vi "Oxford-VRM-Main-Launcher.vi"() -> ()   [LabVIEW 2016]
doc: "This VI will launch the PPMS 2 Instrument backend that will contunously monitor the state of the instrument and log to the DSC. The user has the option of launching a user interface (default) or allowing the backend to run headless. Run \"Launch PPMS2 UI.vi\" here or on a different computer to have a remote user interface. You can also use the APIs like \"Get Temperturature\" interact programmatically with the PPMS 2 Instrument backend."
uses:
  <vilib>/JKI/JKI SMO/SMO/SMO.lvclass
  <vilib>/JKI/JKI SMO/SMO/Typedefs/SMOState --Enum.ctl
  <vilib>/JKI/JKI SMO/SMO.UI/SMO.UI.lvclass
  <userlib>/LevyLab/Levylab Instruments/SMOs/Instrument UI/Instrument UI.lvclass
  SMOs/Instrument.OxfordVRM UI/Instrument.OxfordVRM UI.lvclass
  SMOs/Instrument.OxfordVRM/Instrument.OxfordVRM.lvclass
  C:/Program Files (x86)/National Instruments/LabVIEW 2016/vi.lib/JKI/JKI SMO/SMO/SMO.lvclass
  C:/Program Files (x86)/National Instruments/LabVIEW 2016/user.lib/LevyLab/Levylab Instruments/SMOs/Instrument/Instrument.lvclass
  C:/Program Files (x86)/National Instruments/LabVIEW 2016/vi.lib/JKI/JKI SMO/SMO.UI/SMO.UI.lvclass
  C:/Program Files (x86)/National Instruments/LabVIEW 2016/user.lib/LevyLab/Levylab Instruments/SMOs/Instrument UI/Instrument UI.lvclass
panel:
  in  "Debug Mode?":bool
  in  "Stop":bool=TRUE
  in  "Start":bool=TRUE
  in  "Splash Status":string="Push Start to Start..." caption="String"
  out "UI SMO State":T1=enum."Stopped"
  out "SMO State":T1
  out "error out":errorcluster
  # "OI 1820"
  # "v"
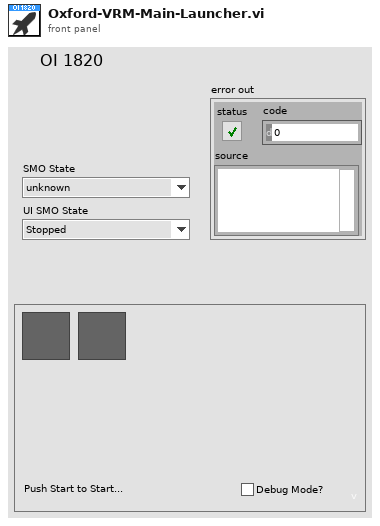
[diagram p1: front panel]
types:
  T1 = typedef "SMO.lvclass/SMOState --Enum.ctl" = enum16{"unknown", "Created", "Started", "Stopped"}
  T2 = enum32{"Invalid", "Standard", "Closed", "Hidden", "Minimized", "Maximized"}
  T3 = enum32{"invalid app kind", "Development System", "Run Time System", "Student Edition", "Embedded LabVIEW", "Evaluation", "Custom"}
  T4 = cluster{"Core":cluster{"Current VI Reference":refnum<vi>, "Close Panel on Exit?":bool}, "Instrument.OxfordVRM":refnum<class "Instrument.OxfordVRM.lvclass">, "Instrument.OxfordVRM UI":refnum<class "Instrument.OxfordVRM UI.lvclass">}
  T5 = cluster{"Current VI Reference":refnum<vi>, "Close Panel on Exit?":bool}
  T6 = typedef "SMO.lvclass/Public Events.ctl" = cluster{"Error":refnum<user-event>, "State":refnum<user-event>, "Reserve State":refnum<user-event>}
  T7 = typedef "SMO.UI.lvclass/PublicEvents--Cluster.ctl" = cluster{"UI Hidden":refnum<user-event>, "UI State":refnum<user-event>}
  T8 = cluster{"Event Registration Refnum":refnum<event-registration>, "Event Registration Refnum":refnum<event-registration>}
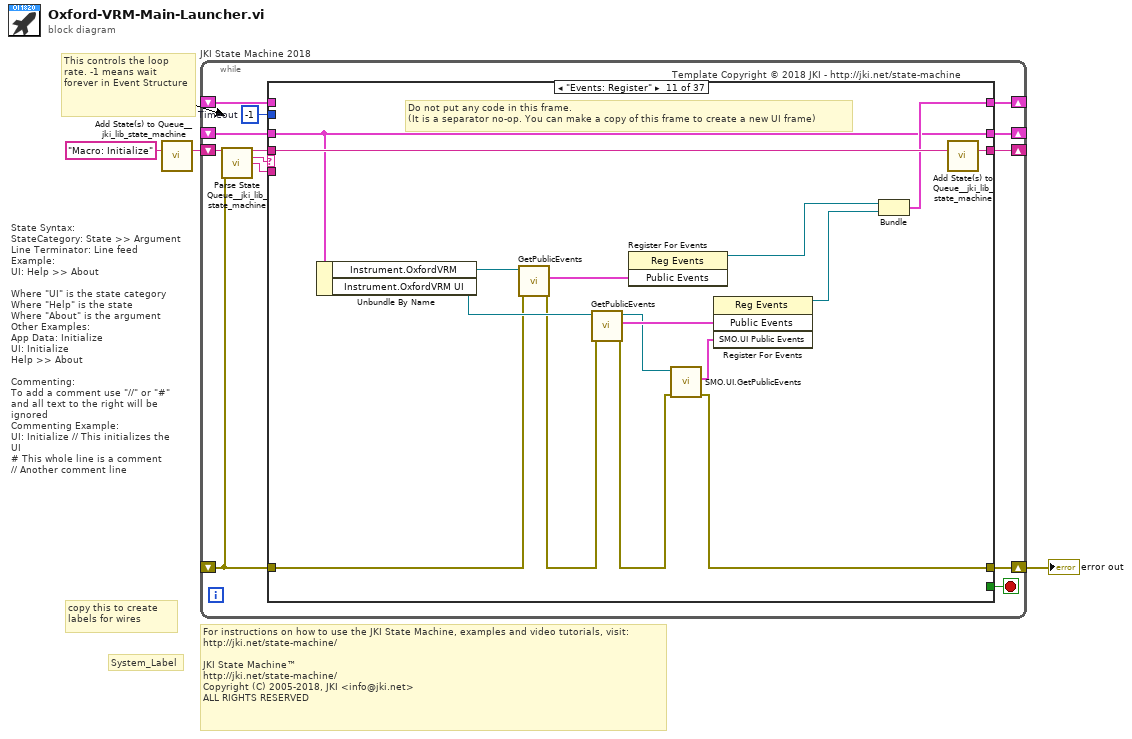
[diagram p0: block diagram]
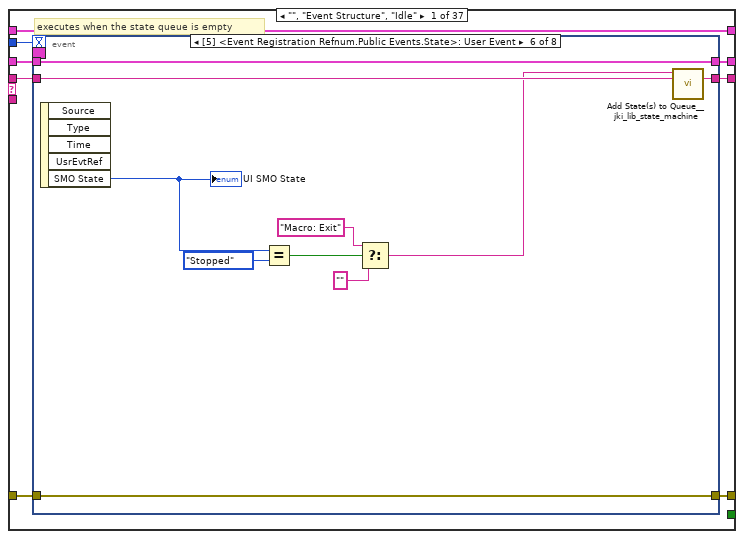
[diagram p2: hidden frame]
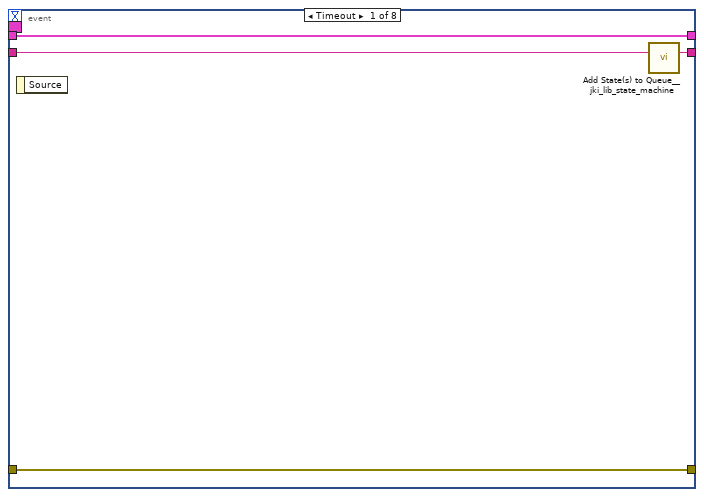
[diagram p3: hidden frame]
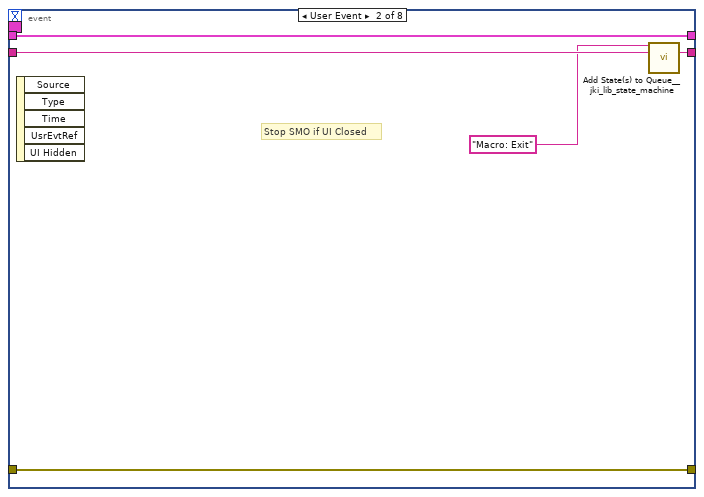
[diagram p4: hidden frame]
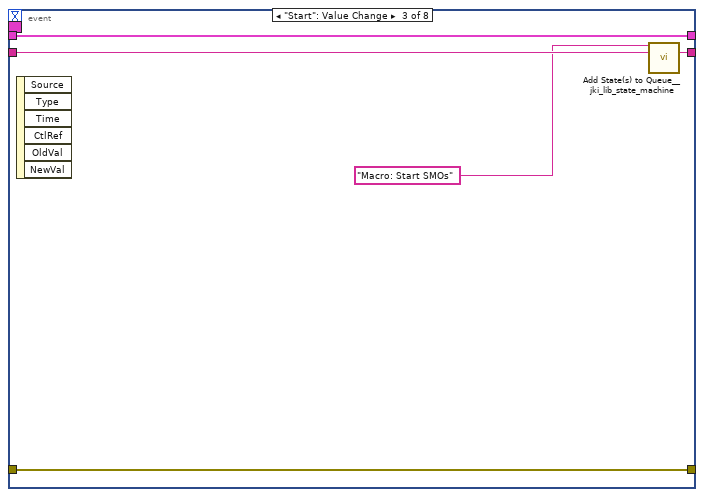
[diagram p5: hidden frame]
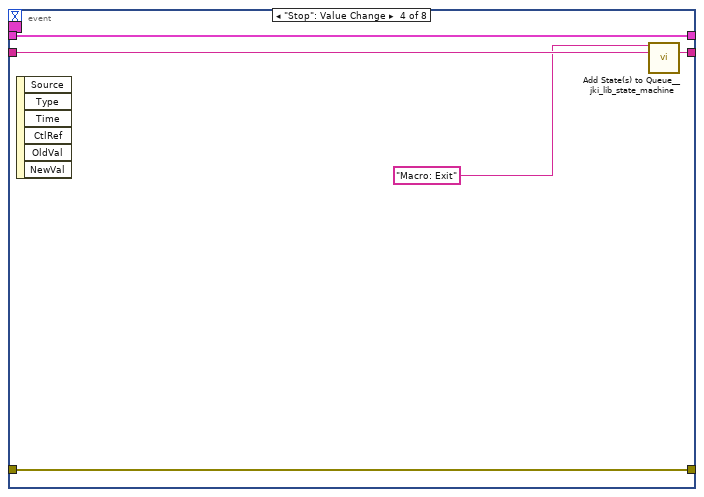
[diagram p6: hidden frame]
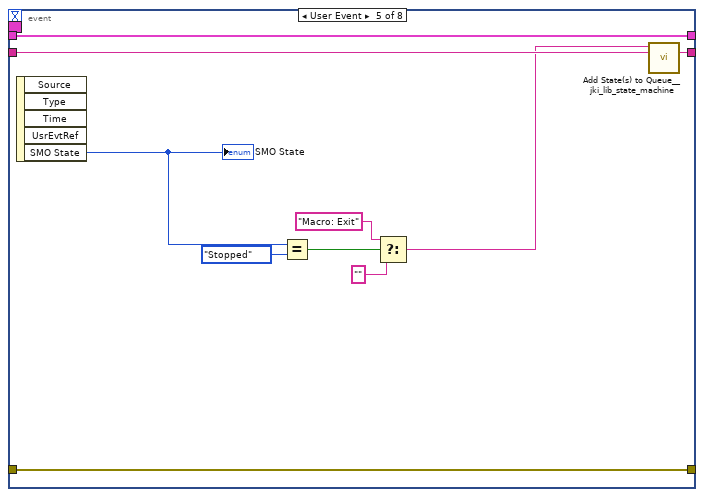
[diagram p7: hidden frame]
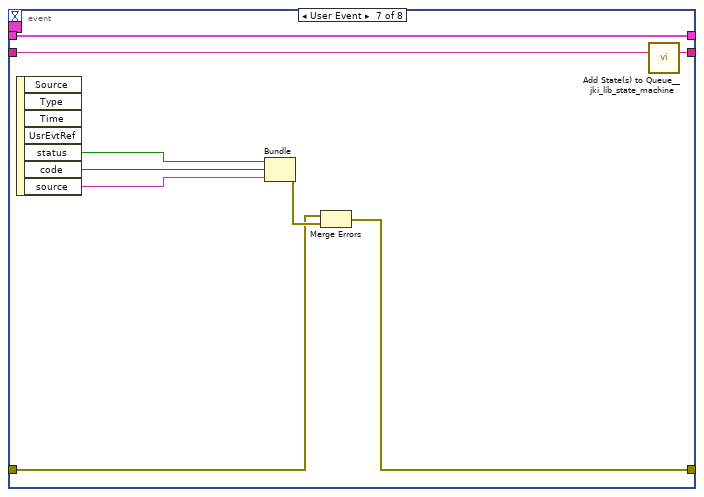
[diagram p8: hidden frame]
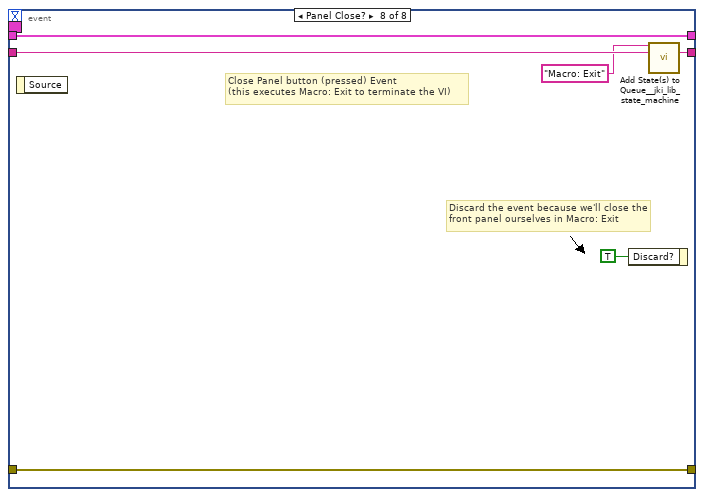
[diagram p9: hidden frame]
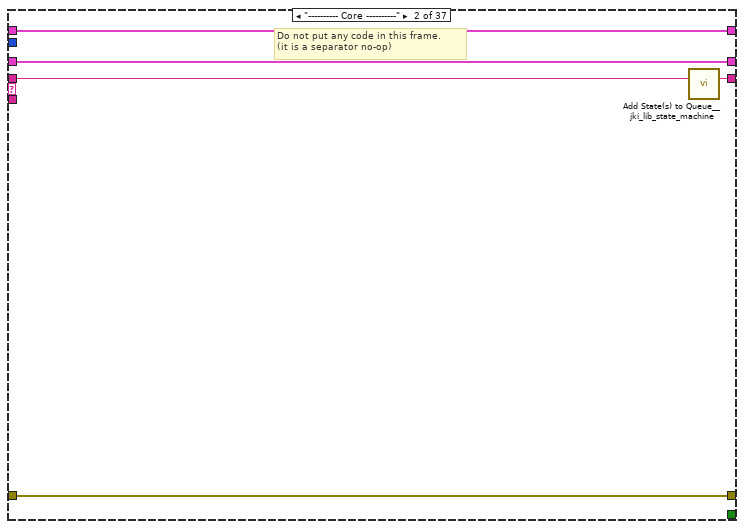
[diagram p10: hidden frame]
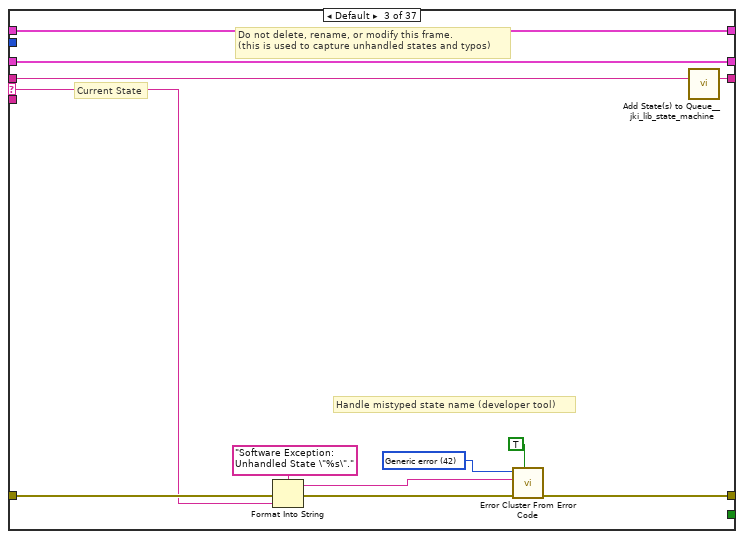
[diagram p11: hidden frame]
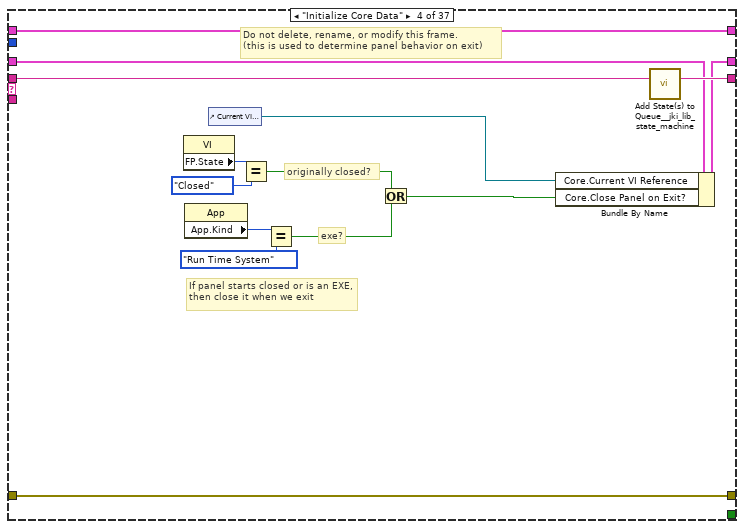
[diagram p12: hidden frame]
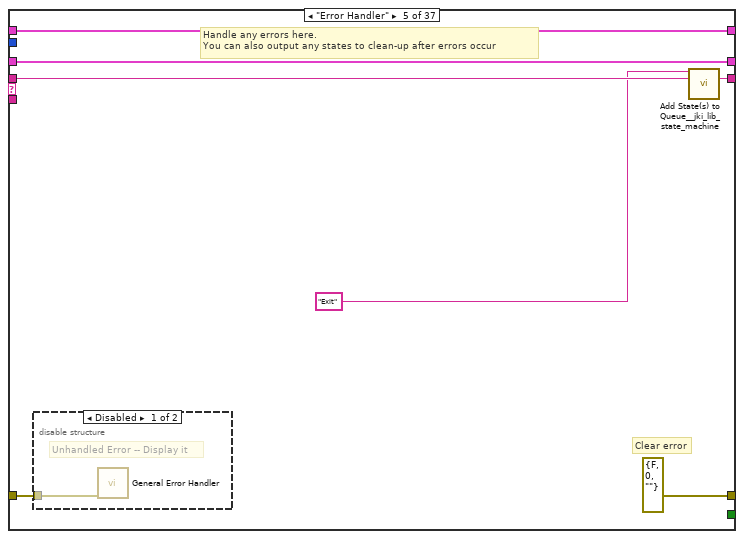
[diagram p13: hidden frame]
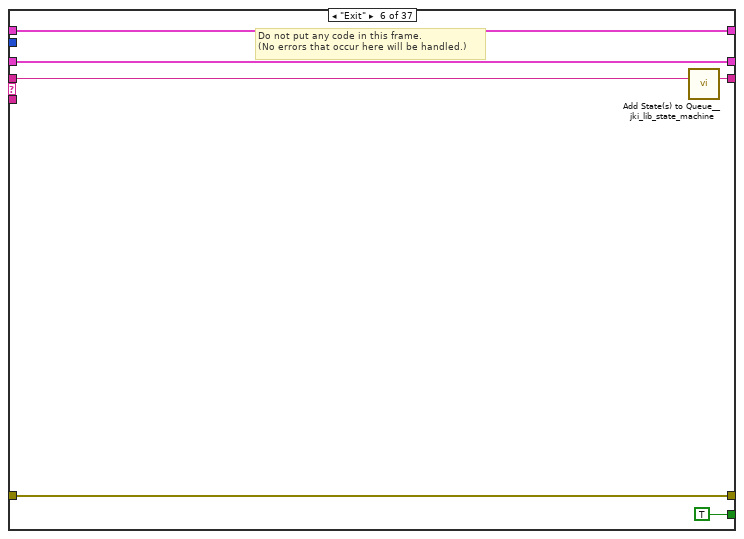
[diagram p15: hidden frame]
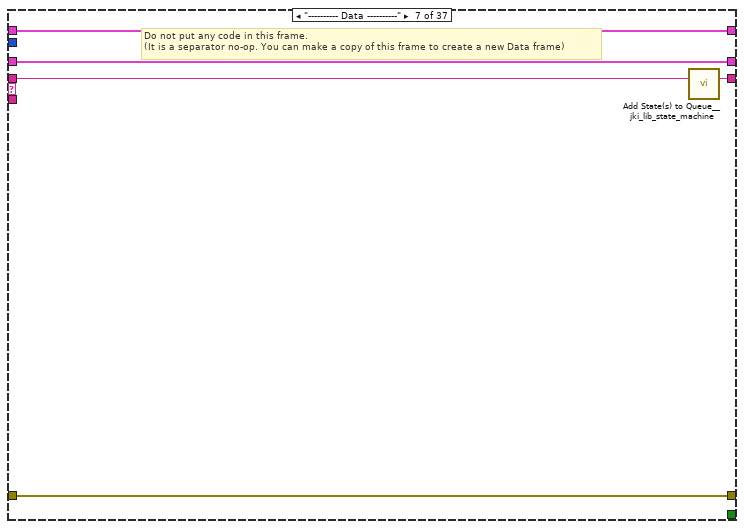
[diagram p16: hidden frame]
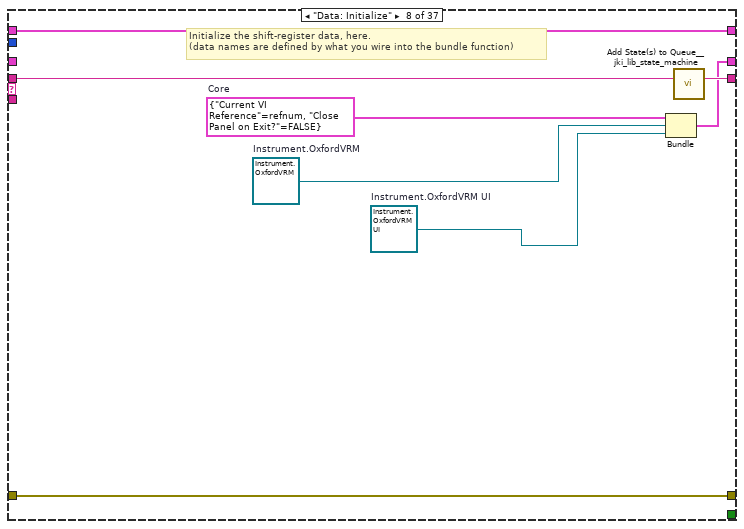
[diagram p17: hidden frame]
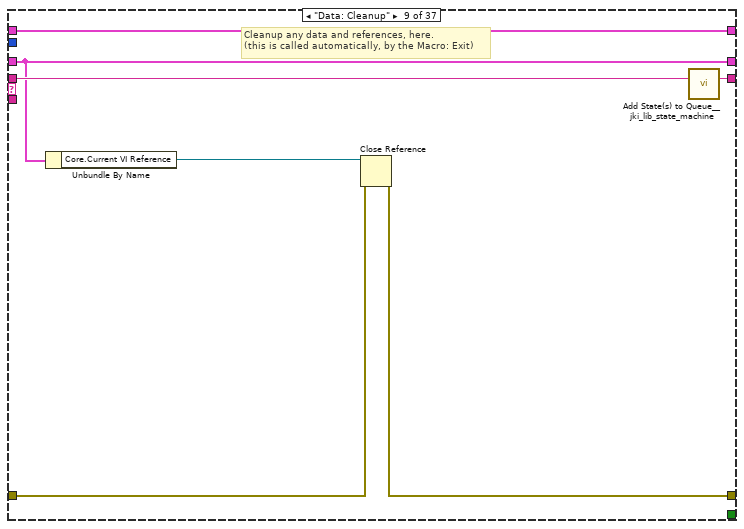
[diagram p18: hidden frame]
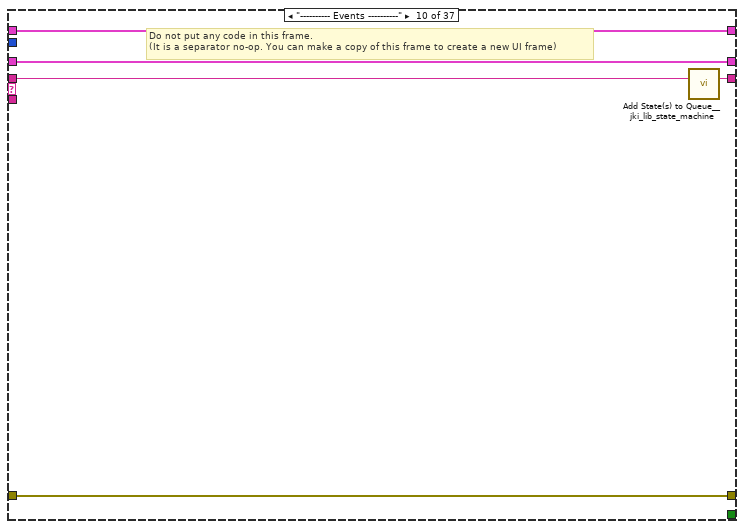
[diagram p19: hidden frame]
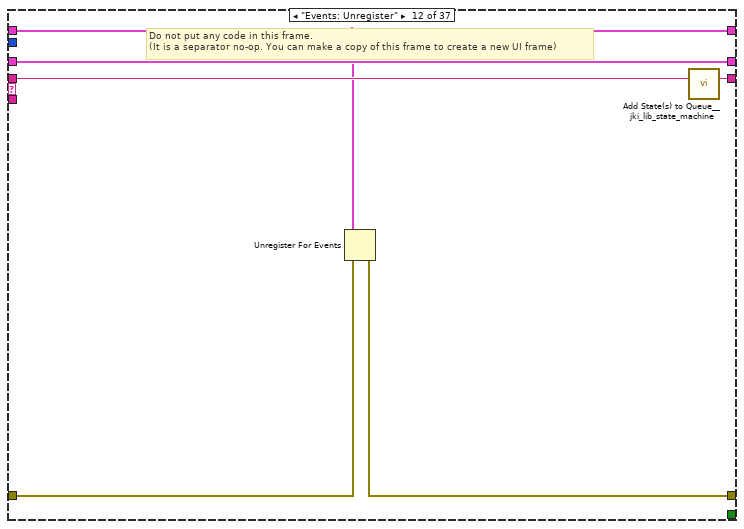
[diagram p20: hidden frame]
diagram:
  # "For instructions on how to use the JKI State Machine, examples and video tutorials, visit:\nhttp://jki.net/state-machine/\n\nJKI State Machine™\nhttp://jki.net/state-machine/\nCopyright (C) 2005-2018, JKI <info@jki.net>\nALL RIGHTS RESERVED"
  # "State Syntax:\nStateCategory: State >> Argument\nLine Terminator: Line feed\nExample:\nUI: Help >> About\n\nWhere \"UI\" is the state category\nWhere \"Help\" is the state\nWhere \"About\" is the argument\nOther Examples:\nApp Data: Initialize\nUI: Initialize\nHelp >> About\n\nCommenting:\nTo add a comment use \"//\" or \"#\" and all text to the right will be ignored\nCommenting Example:\nUI: Initialize // This initializes the UI\n# This whole line is a comment\n// Another comment line"
  # "copy this to create labels for wires"
  # "This controls the loop rate. -1 means wait forever in Event Structure"
  # "System_Label"
  n1 = call <vilib>:"Add State(s) to Queue__jki_lib_state_machine.vi"("State(s) in (\"\")"="Macro: Initialize") -> ("States Out"=w3:string)  [unwired: 14 in]
  n2 = while "JKI State Machine 2018" {
    shift-right: [w9] -> _
    shift-left: _ -> [w4]
    shift-right: [w12] -> w1
    shift-left: _ -> [w7]
    shift-right: [w11] -> _
    shift-left: w3 -> [w13]
    shift-right: [w6] -> _
    shift-left: _ -> [w5]
    stop <- w10 stop-if-true
    w8 = -1  # Timeout
    # "Template Copyright © 2018 JKI - http://jki.net/state-machine"
    n3 = call <vilib>:"Parse State Queue__jki_lib_state_machine.vi"("State Queue"=w13, "Error In (no error)"=w7) -> ("Remaining States"=w15:string, "Current State"=w16:string, "Arguments"=w14:string)  [unwired: 11 in]
    n4 = case shown="\"Events: Register\"" w16 {
      selector: w16 -> [_ _ w85 _ _ _ _ _ _ _ _ _ _ _ _ _ _ _ _ _ _ _ _ _ _ _ _ _ _ _ _ _ _ _ _ _ _]
      tunnel: w15 -> [w24 w83 w89 w109 w116 w123 w128 w136 w143 w148 w164 w170 w175 w181 w188 w200 w278 w283 w288 w294 w300 w306 w318 w323 w337 w346 w357 w372 w386 w393 w404 w419 w434 w449 w458 w465 w470]
      tunnel: w14 -> [_ _ _ _ _ _ _ _ _ _ _ _ _ _ w183 w194 _ _ _ _ _ _ _ _ _ _ _ _ _ _ _ _ _ _ _ w462 _]
      tunnel: [w21 w81 w91 w106 errorcluster {"status"=FALSE, "code"=0, "source"=""} ("error out") w120 w126 w133 w139 w146 w149 w165 w173 w176 w184 w197 w268 w281 w286 w292 w298 w304 w316 w321 w328 w339 w353 w368 w378 w387 w400 w415 w431 w446 w456 w460 w468] -> w12
      tunnel: w7 -> [w20 w81 w90 w106 w112 w120 w126 w133 w140 w146 w155 w166 w173 w178 w185 w198 w269 w281 w286 w292 w298 w304 w316 w321 w331 w340 w349 w364 w379 w388 w397 w412 w429 w442 w456 w461 w468]
      tunnel: [w23 w82 w88 w108 w115 w122 w127 w135 w142 w147 w163 w169 w174 w180 w187 w199 w277 w282 w287 w293 w299 w305 w317 w322 w336 w345 w356 w371 w385 w392 w403 w418 w433 w448 w457 w464 w469] -> w11
      tunnel: [_ _ _ _ _ TRUE _ _ _ _ _ _ _ _ _ _ _ _ _ _ _ _ _ _ _ _ _ _ _ _ _ _ _ _ _ _ _] -> w10
      tunnel: [w19 w80 w87 w107 w113 w121 w125 w134 w138 w145 w158 w168 w172 w179 w186 w196 w266 w280 w285 w291 w297 w303 w315 w320 w334 w341 w354 w369 w382 w390 w401 w416 w430 w445 w455 w463 w467] -> w9
      tunnel: w8 -> [w18 _ _ _ _ _ _ _ _ _ _ _ _ _ _ _ _ _ _ _ _ _ _ _ _ _ _ _ _ _ _ _ _ _ _ _ _]
      tunnel: [w17 w79 w84 w96 w110 w118 w124 w131 w137 w144 w161 w167 w171 w177 w182 w193 w267 w279 w284 w289 w296 w302 w309 w319 w335 w344 w355 w370 w384 w391 w402 w417 w432 w447 w454 w459 w466] -> w6
      tunnel: w5 -> [w17 w79 w84 w96 w110 w118 w124 w131 w137 w144 _ w167 w171 w177 w182 w193 w267 w279 w284 w289 w296 w302 w309 w319 w335 w344 w355 w370 w384 w391 w402 w417 w432 w447 w454 w459 w466]
      tunnel: w4 -> [w22 w80 w87 w102 w113 w121 w125 _ w138 w145 w158 w168 w172 w179 w186 w196 w266 w280 w285 w291 w297 w303 w315 w320 w333 w342 w354 w369 w383 w390 w401 w416 w430 w445 w455 w463 w467]
      frame "", "Event Structure", "Idle" {
        # "executes when the state queue is empty"
        n5 = event shown="[5] <Event Registration Refnum.Public Events.State>: User Event" {
          selector: w17 -> [_ _ _ _ _ _ _ _]
          dyn-events: _ -> [_ _ _ _ _ _ _ _]
          timeout: w18 -> [_ _ _ _ _ _ _ _]
          tunnel: w24 -> [w28 w33 w38 w43 w53 w63 w72 w78]
          tunnel: [w27 w32 w37 w42 w52 w62 w71 w77] -> w23
          tunnel: w22 -> [w25 w30 w35 w40 w50 w60 w70 w75]
          tunnel: [w26 w31 w36 w41 w51 w61 w67 w76] -> w21
          tunnel: w20 -> [w26 w31 w36 w41 w51 w61 w68 w76]
          tunnel: [w25 w30 w35 w40 w50 w60 w70 w75] -> w19
          event Timeout {
            n6 = event-data() -> ()  [unwired: 1 in, 1 out]
            n7 = call <vilib>:"Add State(s) to Queue__jki_lib_state_machine.vi"("State(s) in (\"\")"=w28) -> ("States Out"=w27:string)  [unwired: 14 in]
          }
          event User Event {
            # "Stop SMO if UI Closed"
            n8 = event-data() -> ()  [unwired: 1 in, 5 out]
            n9 = call <vilib>:"Add State(s) to Queue__jki_lib_state_machine.vi"("State(s) in Front (\"\")"="Macro: Exit" ("State(s) in Front (\"\")"), "State(s) in (\"\")"=w33) -> ("States Out"=w32:string)  [unwired: 13 in]
          }
          event "Start": Value Change {
            n10 = event-data() -> ()  [unwired: 1 in, 6 out]
            n11 = call <vilib>:"Add State(s) to Queue__jki_lib_state_machine.vi"("State(s) in Front (\"\")"="Macro: Start SMOs" ("State(s) in Front (\"\")"), "State(s) in (\"\")"=w38) -> ("States Out"=w37:string)  [unwired: 13 in]
          }
          event "Stop": Value Change {
            n12 = event-data() -> ()  [unwired: 1 in, 6 out]
            n13 = call <vilib>:"Add State(s) to Queue__jki_lib_state_machine.vi"("State(s) in Front (\"\")"="Macro: Exit" ("State(s) in Front (\"\")"), "State(s) in (\"\")"=w43) -> ("States Out"=w42:string)  [unwired: 13 in]
          }
          event User Event {
            n14 = event-data() -> ("SMO State"=w45:T1)  [unwired: 1 in, 4 out]
            "SMO State" <- w45
            n15 = Equal?(x=w45, y=SMOState_--Enum."Stopped") -> (x = y?=w48:bool)
            n16 = Select(t="Macro: Exit", s=w48, f="" ("State(s) in Front (\"\")")) -> (s? t:f=w44:string)
            n17 = call <vilib>:"Add State(s) to Queue__jki_lib_state_machine.vi"("State(s) in Front (\"\")"=w44, "State(s) in (\"\")"=w53) -> ("States Out"=w52:string)  [unwired: 13 in]
          }
          event User Event {
            n18 = event-data() -> ("SMO State"=w54:T1)  [unwired: 1 in, 4 out]
            "UI SMO State" <- w54
            n19 = Equal?(x=w54, y=SMOState_--Enum."Stopped") -> (x = y?=w58:bool)
            n20 = Select(t="Macro: Exit", s=w58, f="" ("State(s) in Front (\"\")")) -> (s? t:f=w56:string)
            n21 = call <vilib>:"Add State(s) to Queue__jki_lib_state_machine.vi"("State(s) in Front (\"\")"=w56, "State(s) in (\"\")"=w63) -> ("States Out"=w62:string)  [unwired: 13 in]
          }
          event User Event {
            n22 = event-data() -> ("status"=w64:bool, "code"=w66:i32, "source"=w65:string)  [unwired: 1 in, 4 out]
            n23 = Bundle("status"=w64, "code"=w66, "source"=w65) -> (w69:errorcluster)  [unwired: 1 in]
            n24 = Merge Errors(w68, w69) -> (w67:errorcluster)
            n25 = call <vilib>:"Add State(s) to Queue__jki_lib_state_machine.vi"("State(s) in (\"\")"=w72) -> ("States Out"=w71:string)  [unwired: 14 in]
          }
          event Panel Close? {
            # "Discard the event because we'll close the front panel ourselves in Macro: Exit"
            # "Close Panel button (pressed) Event\n(this executes Macro: Exit to terminate the VI)"
            n26 = event-data() -> ()  [unwired: 1 in, 1 out]
            n27 = event-data("Discard?"=TRUE) -> ()  [unwired: 1 in, 1 out]
            n28 = call <vilib>:"Add State(s) to Queue__jki_lib_state_machine.vi"("State(s) in Front (\"\")"="Macro: Exit", "State(s) in (\"\")"=w78) -> ("States Out"=w77:string)  [unwired: 13 in]
          }
        }
      }
      frame "---------- Core ----------" {
        # "Do not put any code in this frame.\n(it is a separator no-op)"
        n29 = call <vilib>:"Add State(s) to Queue__jki_lib_state_machine.vi"("State(s) in (\"\")"=w83) -> ("States Out"=w82:string)  [unwired: 14 in]
      }
      frame Default {
        w94 = 42 items=["No error", "Argument error", "Memory is full", "Out of zone", "End of file", "File already open", "Generic file I/O error", "File not found", "File permission error", "Disk is full", "Duplicate path", "Too many files open", "System feature not enabled", "Resource file not found", "Cannot add resource", "Resource not found", "Image not found", "Image memory error", "Pen does not exist", "Config type invalid", "Config token not found", "Config parse error", "Config memory error", "Bad external code format", "Bad external code offset", "External code not present", "Null window", "Destroy window error", "Null menu", "Print aborted", "Bad print record", "Print driver error", "Windows error during printing", "Memory error during printing", "Print dialog error", "Generic print error", "Invalid device refnum", "Device not found", "Device parameter error", "Device unit error", "Cannot open device", "Device call aborted", "Generic error", "Cancelled by user", "Object ID too low", "Object ID too high", "Object not in heap", "Unknown heap", "Unknown object (invalid DefProc)", "Unknown object (DefProc not in table)", "Message out of range", "Invalid (null) method", "Unknown message", "Manager call not supported", "Bad address", "Network operation in progress", "Network operation timed out", "Connection is busy", "Network attribute not supported", "Network error", "Address in use", "System out of memory", "Connection aborted", "Connection refused", "Not connected", "Already connected", "Connection closed", "Initialization error (interapplication manager)", "Bad occurrence", "Wait on unbound occurrence handler", "Occurrence queue overflow", "Datalog type conflict", "Unused", "Unrecognized type (interapplication manager)", "Memory corrupt", "Failed to make temporary DLL", "Old CIN version", "Drag socket not found", "Failed to load drop-object", "Failed to register OLE object", "Failed to release OLE object", "Format specifier type mismatch", "Unknown format specifier", "Too few format specifiers", "Too many format specifiers", "Scan failed", "Newer CIN version", "Error converting to variant", "Runtime menu error", "Password tampered", "Variant attribute not found", "Incompatible variant data type", "Event data is not available", "Event Store is not present", "Occurrence is not found", "Event Queue is not created", "Event info is not available", "Refnum passed is NULL", "Error retrieving Class GUID", "Error retrieving CoClass GUID", "Error retrieving TypeLib GUID.", "Bad built application magic bytes.", "Specific driver is different from the specific driver associated with the Logical Name.", "There is no session opened to the class driver.", "Max Error", "MAX - Error with config objects", "MAX - Error loading configuration", "MAX - Group not supported"]
        # "Current State"
        # "Do not delete, rename, or modify this frame.\n(this is used to capture unhandled states and typos)"
        # "Handle mistyped state name (developer tool)"
        n30 = Format Into String(format string="Software Exception: Unhandled State \"%s\"." ("message"), error in=w90, w85) -> (resulting string=w93:string, error out=w92:errorcluster)  [unwired: 1 in]
        n31 = call <vilib>:"Error Cluster From Error Code.vi"("show call chain? (False)"=TRUE, "error in (no error)"=w92, "error message (\"\")"=w93, "error code (0)"=w94) -> ("error out"=w91:errorcluster)  [unwired: 5 in]
        n32 = call <vilib>:"Add State(s) to Queue__jki_lib_state_machine.vi"("State(s) in (\"\")"=w89) -> ("States Out"=w88:string)  [unwired: 14 in]
      }
      frame "Initialize Core Data" {
        # "Do not delete, rename, or modify this frame.\n(this is used to determine panel behavior on exit)"
        # "originally closed?"
        # "exe?"
        # "If panel starts closed or is an EXE, then close it when we exit"
        n33 = property class="VI"() -> ("FP.State"=w99:T2)  [unwired: 2 in, 2 out]
        n34 = property class="App"() -> ("App.Kind"=w105:T3)  [unwired: 2 in, 2 out]
        n35 = control-ref of="Current VI Reference"() -> (w100:refnum<vi>)
        n36 = Equal?(x=w99, y=T2."Closed" ("Front Panel Window:State")) -> (x = y?=w97:bool)
        n37 = Equal?(x=w105, y=T3."Run Time System" ("Application:Kind")) -> (x = y?=w103:bool)
        n38 = Or(x=w97, y=w103) -> (x .or. y?=w101:bool)
        n39 = Bundle By Name(cluster=w102, "Core.Current VI Reference"=w100, "Core.Close Panel on Exit?"=w101) -> (w107:T4)
        n40 = call <vilib>:"Add State(s) to Queue__jki_lib_state_machine.vi"("State(s) in (\"\")"=w109) -> ("States Out"=w108:string)  [unwired: 14 in]
      }
      frame "Error Handler" {
        # "Handle any errors here.\nYou can also output any states to clean-up after errors occur"
        # "Clear error"
        n41 = disable-structure shown="Disabled" {
          disable-tunnel: w112 -> [w117 _]
          frame Disabled {
            # "Unhandled Error -- Display it"
            n42 = call <vilib>:"General Error Handler.vi"("error in (no error)"=w117) -> ()  [unwired: 10 in, 5 out]
          }
          frame Enabled {
          }
        }
        n43 = call <vilib>:"Add State(s) to Queue__jki_lib_state_machine.vi"("State(s) in Front (\"\")"="Exit", "State(s) in (\"\")"=w116) -> ("States Out"=w115:string)  [unwired: 13 in]
      }
      frame "Exit" {
        # "Do not put any code in this frame.\n(No errors that occur here will be handled.)"
        n44 = call <vilib>:"Add State(s) to Queue__jki_lib_state_machine.vi"("State(s) in (\"\")"=w123) -> ("States Out"=w122:string)  [unwired: 14 in]
      }
      frame "---------- Data ----------" {
        # "Do not put any code in this frame.\n(It is a separator no-op. You can make a copy of this frame to create a new Data frame)"
        n45 = call <vilib>:"Add State(s) to Queue__jki_lib_state_machine.vi"("State(s) in (\"\")"=w128) -> ("States Out"=w127:string)  [unwired: 14 in]
      }
      frame "Data: Initialize" {
        w129 = refnum<class "Instrument.OxfordVRM.lvclass"> refnum  # Instrument.OxfordVRM
        w130 = refnum<class "Instrument.OxfordVRM UI.lvclass"> refnum  # Instrument.OxfordVRM UI
        w132 = T5 {"Current VI Reference"=refnum, "Close Panel on Exit?"=FALSE}  # Core
        # "Initialize the shift-register data, here.\n(data names are defined by what you wire into the bundle function)"
        n46 = Bundle("Core"=w132, "Instrument.OxfordVRM"=w129, "Instrument.OxfordVRM UI"=w130) -> (w134:T4)  [unwired: 1 in]
        n47 = call <vilib>:"Add State(s) to Queue__jki_lib_state_machine.vi"("State(s) in (\"\")"=w136) -> ("States Out"=w135:string)  [unwired: 14 in]
      }
      frame "Data: Cleanup" {
        # "Cleanup any data and references, here.\n(this is called automatically, by the Macro: Exit)"
        n48 = Unbundle By Name(w138) -> ("Core.Current VI Reference"=w141:refnum<vi>)
        n49 = Close Reference(reference=w141, error in (no error)=w140) -> (error out=w139:errorcluster)
        n50 = call <vilib>:"Add State(s) to Queue__jki_lib_state_machine.vi"("State(s) in (\"\")"=w143) -> ("States Out"=w142:string)  [unwired: 14 in]
      }
      frame "---------- Events ----------" {
        # "Do not put any code in this frame.\n(It is a separator no-op. You can make a copy of this frame to create a new UI frame)"
        n51 = call <vilib>:"Add State(s) to Queue__jki_lib_state_machine.vi"("State(s) in (\"\")"=w148) -> ("States Out"=w147:string)  [unwired: 14 in]
      }
      frame "Events: Register" {
        # "Do not put any code in this frame.\n(It is a separator no-op. You can make a copy of this frame to create a new UI frame)"
        n52 = Unbundle By Name(w158) -> ("Instrument.OxfordVRM"=w157:refnum<class "Instrument.OxfordVRM.lvclass">, "Instrument.OxfordVRM UI"=w156:refnum<class "Instrument.OxfordVRM UI.lvclass">)
        n53 = call <vilib>:"GetPublicEvents.vi"("error in (no error)"=w155, "SMO"=w157) -> ("error out"=w154:errorcluster, "Public Events"=w159:T6)  [unwired: 7 in, 1 out]
        n54 = call <vilib>:"GetPublicEvents.vi"("error in (no error)"=w154, "SMO"=w156) -> ("error out"=w150:errorcluster, "Public Events"=w160:T6, "SMO out"=w152:refnum<class "Instrument.OxfordVRM UI.lvclass">)  [unwired: 7 in]
        n55 = register-events(w159) -> (reference out=w162:refnum<event-registration>)  [unwired: 2 in, 1 out]
        n56 = call <vilib>:"SMO.UI.GetPublicEvents.vi"("error in (no error)"=w150, "SMO.UI"=w152) -> ("error out"=w149:errorcluster, "SMO.UI Public Events"=w151:T7)  [unwired: 7 in, 1 out]
        n57 = register-events(w160, w151) -> (reference out=w153:refnum<event-registration>)  [unwired: 2 in, 1 out]
        n58 = Bundle("Event Registration Refnum"=w162, "Event Registration Refnum"=w153) -> (w161:T8)  [unwired: 1 in]
        n59 = call <vilib>:"Add State(s) to Queue__jki_lib_state_machine.vi"("State(s) in (\"\")"=w164) -> ("States Out"=w163:string)  [unwired: 14 in]
      }
      frame "Events: Unregister" {
        # "Do not put any code in this frame.\n(It is a separator no-op. You can make a copy of this frame to create a new UI frame)"
        n60 = Unregister For Events(event registration refnum=w167, error in=w166) -> (error out=w165:errorcluster)
        n61 = call <vilib>:"Add State(s) to Queue__jki_lib_state_machine.vi"("State(s) in (\"\")"=w170) -> ("States Out"=w169:string)  [unwired: 14 in]
      }
      frame "---------- UI ----------" {
        # "Do not put any code in this frame.\n(It is a separator no-op. You can make a copy of this frame to create a new UI frame)"
        n62 = call <vilib>:"Add State(s) to Queue__jki_lib_state_machine.vi"("State(s) in (\"\")"=w175) -> ("States Out"=w174:string)  [unwired: 14 in]
      }
      frame "UI: Initialize" {
        # "Initialize the User Interface, here.\n(this is called automatically, by the Macro: Init)"
        n63 = invoke on="Stop" class="Bool (strict)" method="Reinit To Default"() -> ()  [unwired: 3 in, 3 out]
        n64 = invoke on="error out" class="Clust (strict)" method="Reinit To Default"() -> ()  [unwired: 3 in, 3 out]
        n65 = invoke on="SMO State" class="Enum (strict)" method="Reinit To Default"() -> ()  [unwired: 3 in, 3 out]
        n66 = invoke on="Start" class="Bool (strict)" method="Reinit To Default"() -> ()  [unwired: 3 in, 3 out]
        n67 = call <userlib>:"Fit VI window to Largest Dec__ogtk.vi"("error in (no error)"=w178) -> ("error out"=w176:errorcluster)  [unwired: 5 in, 1 out]
        n68 = call <vilib>:"Add State(s) to Queue__jki_lib_state_machine.vi"("State(s) in (\"\")"=w181) -> ("States Out"=w180:string)  [unwired: 14 in]
      }
      frame "UI: Cursor Set" {
        # "Argument"
        # "Set and Unset Cursor Busy.\n(Usage: \"UI: Cursor Set >> Busy|Idle\")"
        n69 = case shown="\"Idle\", Default" w183 {
          tunnel: w185 -> [w190 w192]
          tunnel: [w189 w191] -> w184
          frame "Idle", Default {
            n70 = call <vilib>:"Unset Busy.vi"("error in (no error)"=w190) -> ("error out"=w189:errorcluster)  [unwired: 10 in]
          }
          frame "Busy" {
            n71 = call <vilib>:"Set Busy.vi"("error in (no error)"=w192) -> ("error out"=w191:errorcluster)  [unwired: 9 in, 1 out]
          }
        }
        n72 = call <vilib>:"Add State(s) to Queue__jki_lib_state_machine.vi"("State(s) in (\"\")"=w188) -> ("States Out"=w187:string)  [unwired: 14 in]
      }
      frame "UI: Front Panel State" {
        # "Argument"
        # "Set Front Panel Open or Closed\n(Usage: \"UI: Front Panel State >> Open|Close\")"
        n73 = Unbundle By Name(w196) -> ("Core.Current VI Reference"=w195:refnum<vi>)
        n74 = case shown="\"Open\", \"Standard\", Default" w194 {
          tunnel: w198 -> [w206 w221 w232 w245 w258]
          tunnel: [w208 w222 w234 w247 w260] -> w197
          tunnel: w195 -> [w207 w219 w233 w246 w259]
          frame "Open", "Standard", Default {
            w201 = T2."Standard" ("State")
            n75 = property class="VI"(reference=w207, error in=w206) -> (reference out=w204:refnum<vi>, error out=w205:errorcluster, "FP.State"=w203:T2)
            n76 = Not Equal?(x=w203, y=w201) -> (x != y?=w202:bool)
            n77 = case shown="False" w202 {
              tunnel: [w212 w214] -> w208
              tunnel: w205 -> [w211 w214]
              tunnel: w204 -> [w210 _]
              tunnel: w201 -> [w209 _]
              frame True {
                n78 = invoke class="VI" method="FP.Open"(reference=w210, error in=w211, "Activate"=TRUE, "State"=w209) -> (error out=w212:errorcluster)  [unwired: 1 in, 4 out]
              }
              frame False {
              }
            }
          }
          frame "Close", "Closed" {
            n79 = property class="VI"(reference=w219, error in=w221) -> (reference out=w218:refnum<vi>, error out=w220:errorcluster, "FP.State"=w216:T2)
            n80 = Not Equal?(x=w216, y=T2."Closed" ("Front Panel Window:State")) -> (x != y?=w215:bool)
            n81 = case shown="True" w215 {
              tunnel: [w223 w226] -> w222
              tunnel: w220 -> [w223 w225]
              tunnel: w218 -> [_ w224]
              frame False {
              }
              frame True {
                n82 = invoke class="VI" method="FP.Close"(reference=w224, error in=w225) -> (error out=w226:errorcluster)  [unwired: 1 in, 2 out]
              }
            }
          }
          frame "Hidden", "Hide" {
            w227 = T2."Hidden" ("State")
            n83 = property class="VI"(reference=w233, error in=w232) -> (reference out=w230:refnum<vi>, error out=w231:errorcluster, "FP.State"=w229:T2)
            n84 = Not Equal?(x=w229, y=w227) -> (x != y?=w228:bool)
            n85 = case shown="True" w228 {
              tunnel: [w238 w239] -> w234
              tunnel: w231 -> [w237 w239]
              tunnel: w230 -> [w236 _]
              tunnel: w227 -> [w235 _]
              frame True {
                n86 = invoke class="VI" method="FP.Open"(reference=w236, error in=w237, "State"=w235) -> (error out=w238:errorcluster)  [unwired: 2 in, 4 out]
              }
              frame False {
              }
            }
          }
          frame "Minimize", "Minimized" {
            w240 = T2."Minimized" ("State")
            n87 = property class="VI"(reference=w246, error in=w245) -> (reference out=w243:refnum<vi>, error out=w244:errorcluster, "FP.State"=w242:T2)
            n88 = Not Equal?(x=w242, y=w240) -> (x != y?=w241:bool)
            n89 = case shown="True" w241 {
              tunnel: [w251 w252] -> w247
              tunnel: w244 -> [w250 w252]
              tunnel: w243 -> [w249 _]
              tunnel: w240 -> [w248 _]
              frame True {
                n90 = invoke class="VI" method="FP.Open"(reference=w249, error in=w250, "State"=w248) -> (error out=w251:errorcluster)  [unwired: 2 in, 4 out]
              }
              frame False {
              }
            }
          }
          frame "Maximize", "Maximized" {
            w253 = T2."Maximized" ("State")
            n91 = property class="VI"(reference=w259, error in=w258) -> (reference out=w256:refnum<vi>, error out=w257:errorcluster, "FP.State"=w255:T2)
            n92 = Not Equal?(x=w255, y=w253) -> (x != y?=w254:bool)
            n93 = case shown="True" w254 {
              tunnel: [w264 w265] -> w260
              tunnel: w257 -> [w263 w265]
              tunnel: w256 -> [w262 _]
              tunnel: w253 -> [w261 _]
              frame True {
                n94 = invoke class="VI" method="FP.Open"(reference=w262, error in=w263, "State"=w261) -> (error out=w264:errorcluster)  [unwired: 2 in, 4 out]
              }
              frame False {
              }
            }
          }
        }
        n95 = call <vilib>:"Add State(s) to Queue__jki_lib_state_machine.vi"("State(s) in (\"\")"=w200) -> ("States Out"=w199:string)  [unwired: 14 in]
      }
      frame "UI: Set Background Color" {
        # "Do not put any code in this frame.\n(It is a separator no-op. You can make a copy of this frame to create a new UI frame)"
        n96 = property class="VI"(error in=w269) -> (error out=w271:errorcluster, "Panel"=w272:refnum<vi>)  [unwired: 1 in, 1 out]
        n97 = property class="Pnl"(reference=w272, error in=w271) -> (error out=w270:errorcluster, "Panes[]"=w273:refnum<vi>[])  [unwired: 1 out]
        n98 = Index Array(array=w273, index=0) -> (element=w275:refnum<vi>)
        n99 = property class="Pane"(reference=w275, error in=w270, "PaneColor"=u32 16777238 ("Color Box")) -> (error out=w268:errorcluster)  [unwired: 1 out]
        n100 = call <vilib>:"Add State(s) to Queue__jki_lib_state_machine.vi"("State(s) in (\"\")"=w278) -> ("States Out"=w277:string)  [unwired: 14 in]
      }
      frame "UI: Exit" {
        # "Do not put any code in this frame.\n(It is a separator no-op. You can make a copy of this frame to create a new UI frame)"
        n101 = invoke on="Start" class="Bool (strict)" method="Reinit To Default"() -> ()  [unwired: 3 in, 3 out]
        n102 = invoke on="Stop" class="Bool (strict)" method="Reinit To Default"() -> ()  [unwired: 3 in, 3 out]
        n103 = call <vilib>:"Add State(s) to Queue__jki_lib_state_machine.vi"("State(s) in (\"\")"=w283) -> ("States Out"=w282:string)  [unwired: 14 in]
      }
      frame "---------- Macro ----------" {
        # "Do not put any code in this frame.\n(It is a separator no-op. You can make a copy of this frame to create a new Macro frame)"
        n104 = call <vilib>:"Add State(s) to Queue__jki_lib_state_machine.vi"("State(s) in (\"\")"=w288) -> ("States Out"=w287:string)  [unwired: 14 in]
      }
      frame "Macro: Initialize" {
        # "Initialization Macro\n(This is called once, when the VI starts)"
        n105 = call <vilib>:"Add State(s) to Queue__jki_lib_state_machine.vi"("State(s) in Front (\"\")"="Data: Initialize\nInitialize Core Data\n//Events: Register\nUI: Initialize\nUI: Front Panel State >> Open\nUI: Set Background Color\nSplash: Set Status >> Push Start to Start...", "State(s) in (\"\")"=w294) -> ("States Out"=w293:string)  [unwired: 13 in]
      }
      frame "Macro: Start SMOs" {
        # "Do not put any code in this frame.\n(It is a separator no-op. You can make a copy of this frame to create a new Macro frame)"
        n106 = call <vilib>:"Add State(s) to Queue__jki_lib_state_machine.vi"("State(s) in Front (\"\")"="Splash: Set Status >> Starting Instrument...\nSMO: Create Instrument\nSMO: Create Instrument UI\nEvents: Register\nSMO: Start Instrument\nSplash: Set Status >> Instrument Process Started...\nSplash: Set Status >> Starting User Interface...\nSMO: Start Instrument UI\nUI: Front Panel State >> Hide\nSMO: Show Instrument UI" ("State(s) in Front (\"\")"), "State(s) in (\"\")"=w300) -> ("States Out"=w299:string)  [unwired: 13 in]
      }
      frame "Macro: Stop SMOs" {
        # "Do not put any code in this frame.\n(It is a separator no-op. You can make a copy of this frame to create a new Macro frame)"
        n107 = call <vilib>:"Add State(s) to Queue__jki_lib_state_machine.vi"("State(s) in Front (\"\")"="SMO: Stop Instrument\nSMO: Destroy Instrument\nSMO: Hide Instrument UI\nSMO: Stop Instrument UI\nSMO: Destroy Instrument UI" ("State(s) in Front (\"\")"), "State(s) in (\"\")"=w306) -> ("States Out"=w305:string)  [unwired: 13 in]
      }
      frame "Macro: Exit" {
        # "Exit Macro\n(This is called once, when the VI exits)"
        n108 = Unbundle By Name(w315) -> ("Core.Close Panel on Exit?"=w314:bool)
        n109 = Select(t="UI: Front Panel State >> Open", s=w314, f="") -> (s? t:f=w311:string)
        n110 = call <vilib>:"Add State(s) to Queue__jki_lib_state_machine.vi"("State(s) in Front (\"\")"="UI: Front Panel State >> Open\nUI: Exit", "State(s) in (\"\")"=w311, "State(s) at Back (\"\")"="Macro: Stop SMOs\nData: Cleanup\nEvents: Unregister\nExit") -> ("States Out"=w310:string)  [unwired: 12 in]
        n111 = call <vilib>:"Add State(s) to Queue__jki_lib_state_machine.vi"("State(s) in Front (\"\")"=w310, "State(s) in (\"\")"=w318) -> ("States Out"=w317:string)  [unwired: 13 in]
      }
      frame "---------- SMO ----------" {
        # "Do not put any code in this frame.\n(It is a separator no-op. You can make a copy of this frame to create a new Macro frame)"
        n112 = call <vilib>:"Add State(s) to Queue__jki_lib_state_machine.vi"("State(s) in (\"\")"=w323) -> ("States Out"=w322:string)  [unwired: 14 in]
      }
      frame "SMO: Create Instrument" {
        # "Do not put any code in this frame.\n(It is a separator no-op. You can make a copy of this frame to create a new Macro frame)"
        n113 = Unbundle By Name(w333) -> ("Instrument.OxfordVRM"=w332:refnum<class "Instrument.OxfordVRM.lvclass">)
        n114 = call-dynamic "Create Instrument SMO.vi"("error in (no error)"=w331, "Debug Mode? [F]"="Debug Mode?", "Configuration Window? [T]"=FALSE, "Instrument in"=w332) -> ("error out"=w325:errorcluster, "Instrument out"=w329:refnum<class "Instrument.OxfordVRM.lvclass">)  [unwired: 6 in]
        n115 = call-dynamic "Write Data Logger.vi"("error in (no error)"=w325, "Data Logger"=enum16{"DSC", "PGSQL"}."PGSQL", "Instrument in"=w329) -> ("error out"=w328:errorcluster, "Instrument out"=w324:refnum<class "Instrument.OxfordVRM.lvclass">)  [unwired: 7 in]
        n116 = Bundle By Name(cluster=w333, "Instrument.OxfordVRM"=w324) -> (w334:T4)
        n117 = call <vilib>:"Add State(s) to Queue__jki_lib_state_machine.vi"("State(s) in (\"\")"=w337) -> ("States Out"=w336:string)  [unwired: 14 in]
      }
      frame "SMO: Start Instrument" {
        # "Do not put any code in this frame.\n(It is a separator no-op. You can make a copy of this frame to create a new Macro frame)"
        n118 = Unbundle By Name(w342) -> ("Instrument.OxfordVRM"=w343:refnum<class "Instrument.OxfordVRM.lvclass">)
        n119 = call <vilib>:"Start.vi"("error in (no error)"=w340, "SMO"=w343) -> ("error out"=w339:errorcluster, "SMO out"=w338:refnum<class "Instrument.OxfordVRM.lvclass">)  [unwired: 8 in]
        n120 = Bundle By Name(cluster=w342, "Instrument.OxfordVRM"=w338) -> (w341:T4)
        n121 = call <vilib>:"Add State(s) to Queue__jki_lib_state_machine.vi"("State(s) in (\"\")"=w346) -> ("States Out"=w345:string)  [unwired: 14 in]
      }
      frame "SMO: Stop Instrument" {
        # "Do not put any code in this frame.\n(It is a separator no-op. You can make a copy of this frame to create a new Macro frame)"
        n122 = Unbundle By Name(w354) -> ("Instrument.OxfordVRM"=w352:refnum<class "Instrument.OxfordVRM.lvclass">)
        n123 = call <vilib>:"GetState.vi"("error in (no error)"=w349, "SMO"=w352) -> ("error out"=w348:errorcluster, "SMO State"=w351:T1, "SMO out"=w347:refnum<class "Instrument.OxfordVRM.lvclass">)  [unwired: 7 in]
        n124 = call <vilib>:"Clear Errors.vi"("error in (no error)"=w348) -> ("error out"=w350:errorcluster)  [unwired: 5 in, 1 out]
        n125 = case shown="\"Created\", \"Started\"" w351 {
          tunnel: [w358 w361] -> w353
          tunnel: w350 -> [w358 w360]
          tunnel: w347 -> [_ w359]
          frame Default {
          }
          frame "Created", "Started" {
            n126 = call <vilib>:"Stop.vi"("error in (no error)"=w360, "SMO"=w359) -> ("error out"=w361:errorcluster)  [unwired: 8 in, 1 out]
          }
        }
        n127 = call <vilib>:"Add State(s) to Queue__jki_lib_state_machine.vi"("State(s) in (\"\")"=w357) -> ("States Out"=w356:string)  [unwired: 14 in]
      }
      frame "SMO: Destroy Instrument" {
        # "Do not put any code in this frame.\n(It is a separator no-op. You can make a copy of this frame to create a new Macro frame)"
        n128 = Unbundle By Name(w369) -> ("Instrument.OxfordVRM"=w367:refnum<class "Instrument.OxfordVRM.lvclass">)
        n129 = call <vilib>:"GetState.vi"("error in (no error)"=w364, "SMO"=w367) -> ("error out"=w363:errorcluster, "SMO State"=w366:T1, "SMO out"=w362:refnum<class "Instrument.OxfordVRM.lvclass">)  [unwired: 7 in]
        n130 = call <vilib>:"Clear Errors.vi"("error in (no error)"=w363) -> ("error out"=w365:errorcluster)  [unwired: 5 in, 1 out]
        n131 = case shown="\"Stopped\"" w366 {
          tunnel: [w373 w376] -> w368
          tunnel: w365 -> [w373 w375]
          tunnel: w362 -> [_ w374]
          frame Default {
          }
          frame "Stopped" {
            n132 = call <vilib>:"Destroy.vi"("error in (no error)"=w375, "SMO"=w374) -> ("error out"=w376:errorcluster)  [unwired: 9 in]
          }
        }
        n133 = call <vilib>:"Add State(s) to Queue__jki_lib_state_machine.vi"("State(s) in (\"\")"=w372) -> ("States Out"=w371:string)  [unwired: 14 in]
      }
      frame "SMO: Create Instrument UI" {
        # "Do not put any code in this frame.\n(It is a separator no-op. You can make a copy of this frame to create a new Macro frame)"
        n134 = Unbundle By Name(w383) -> ("Instrument.OxfordVRM UI"=w381:refnum<class "Instrument.OxfordVRM UI.lvclass">, "Instrument.OxfordVRM"=w377:refnum<class "Instrument.OxfordVRM.lvclass">)
        n135 = call <userlib>:"Create UI.vi"("error in (no error)"=w379, "Instrument in"=w377, "Instrument UI"=w381) -> ("error out"=w378:errorcluster, "Instrument UI out"=w380:refnum<class "Instrument.OxfordVRM UI.lvclass">)  [unwired: 7 in]
        n136 = Bundle By Name(cluster=w383, "Instrument.OxfordVRM UI"=w380) -> (w382:T4)
        n137 = call <vilib>:"Add State(s) to Queue__jki_lib_state_machine.vi"("State(s) in (\"\")"=w386) -> ("States Out"=w385:string)  [unwired: 14 in]
      }
      frame "SMO: Start Instrument UI" {
        # "Do not put any code in this frame.\n(It is a separator no-op. You can make a copy of this frame to create a new Macro frame)"
        n138 = Unbundle By Name(w390) -> ("Instrument.OxfordVRM UI"=w389:refnum<class "Instrument.OxfordVRM UI.lvclass">)
        n139 = call <vilib>:"Start.vi"("error in (no error)"=w388, "SMO"=w389) -> ("error out"=w387:errorcluster)  [unwired: 8 in, 1 out]
        n140 = call <vilib>:"Add State(s) to Queue__jki_lib_state_machine.vi"("State(s) in (\"\")"=w393) -> ("States Out"=w392:string)  [unwired: 14 in]
      }
      frame "SMO: Show Instrument UI" {
        # "Do not put any code in this frame.\n(It is a separator no-op. You can make a copy of this frame to create a new Macro frame)"
        n141 = Unbundle By Name(w401) -> ("Instrument.OxfordVRM UI"=w399:refnum<class "Instrument.OxfordVRM UI.lvclass">)
        n142 = call <vilib>:"GetState.vi"("error in (no error)"=w397, "SMO"=w399) -> ("error out"=w395:errorcluster, "SMO State"=w394:T1, "SMO out"=w398:refnum<class "Instrument.OxfordVRM UI.lvclass">)  [unwired: 7 in]
        n143 = call <vilib>:"Clear Errors.vi"("error in (no error)"=w395) -> ("error out"=w396:errorcluster)  [unwired: 5 in, 1 out]
        n144 = case shown="\"Started\"" w394 {
          tunnel: [w405 w408] -> w400
          tunnel: w398 -> [_ w407]
          tunnel: w396 -> [w405 w406]
          frame Default {
          }
          frame "Started" {
            n145 = call <vilib>:"Show.vi"("error in (no error)"=w406, "SMO.UI"=w407) -> ("error out"=w408:errorcluster)  [unwired: 8 in, 1 out]
          }
        }
        n146 = call <vilib>:"Add State(s) to Queue__jki_lib_state_machine.vi"("State(s) in (\"\")"=w404) -> ("States Out"=w403:string)  [unwired: 14 in]
      }
      frame "SMO: Hide Instrument UI" {
        # "Do not put any code in this frame.\n(It is a separator no-op. You can make a copy of this frame to create a new Macro frame)"
        n147 = Unbundle By Name(w416) -> ("Instrument.OxfordVRM UI"=w414:refnum<class "Instrument.OxfordVRM UI.lvclass">)
        n148 = call <vilib>:"GetState.vi"("error in (no error)"=w412, "SMO"=w414) -> ("error out"=w410:errorcluster, "SMO State"=w409:T1, "SMO out"=w413:refnum<class "Instrument.OxfordVRM UI.lvclass">)  [unwired: 7 in]
        n149 = call <vilib>:"Clear Errors.vi"("error in (no error)"=w410) -> ("error out"=w411:errorcluster)  [unwired: 5 in, 1 out]
        n150 = case shown="\"Started\"" w409 {
          tunnel: [w420 w423] -> w415
          tunnel: w413 -> [_ w422]
          tunnel: w411 -> [w420 w421]
          frame Default {
          }
          frame "Started" {
            n151 = call <vilib>:"Hide.vi"("error in (no error)"=w421, "SMO.UI"=w422) -> ("error out"=w423:errorcluster)  [unwired: 8 in, 1 out]
          }
        }
        n152 = call <vilib>:"Add State(s) to Queue__jki_lib_state_machine.vi"("State(s) in (\"\")"=w419) -> ("States Out"=w418:string)  [unwired: 14 in]
      }
      frame "SMO: Stop Instrument UI" {
        # "Do not put any code in this frame.\n(It is a separator no-op. You can make a copy of this frame to create a new Macro frame)"
        n153 = Unbundle By Name(w430) -> ("Instrument.OxfordVRM UI"=w425:refnum<class "Instrument.OxfordVRM UI.lvclass">)
        n154 = call <vilib>:"GetState.vi"("error in (no error)"=w429, "SMO"=w425) -> ("error out"=w428:errorcluster, "SMO State"=w426:T1, "SMO out"=w424:refnum<class "Instrument.OxfordVRM UI.lvclass">)  [unwired: 7 in]
        n155 = call <vilib>:"Clear Errors.vi"("error in (no error)"=w428) -> ("error out"=w427:errorcluster)  [unwired: 5 in, 1 out]
        n156 = case shown="\"Created\", \"Started\"" w426 {
          tunnel: [w435 w438] -> w431
          tunnel: w424 -> [_ w437]
          tunnel: w427 -> [w435 w436]
          frame Default {
          }
          frame "Created", "Started" {
            n157 = call <vilib>:"Stop.vi"("error in (no error)"=w436, "SMO"=w437) -> ("error out"=w438:errorcluster)  [unwired: 8 in, 1 out]
          }
        }
        n158 = call <vilib>:"Add State(s) to Queue__jki_lib_state_machine.vi"("State(s) in (\"\")"=w434) -> ("States Out"=w433:string)  [unwired: 14 in]
      }
      frame "SMO: Destroy Instrument UI" {
        # "Do not put any code in this frame.\n(It is a separator no-op. You can make a copy of this frame to create a new Macro frame)"
        n159 = Unbundle By Name(w445) -> ("Instrument.OxfordVRM UI"=w444:refnum<class "Instrument.OxfordVRM UI.lvclass">)
        n160 = call <vilib>:"GetState.vi"("error in (no error)"=w442, "SMO"=w444) -> ("error out"=w441:errorcluster, "SMO State"=w439:T1, "SMO out"=w443:refnum<class "Instrument.OxfordVRM UI.lvclass">)  [unwired: 7 in]
        n161 = call <vilib>:"Clear Errors.vi"("error in (no error)"=w441) -> ("error out"=w440:errorcluster)  [unwired: 5 in, 1 out]
        n162 = case shown="\"Stopped\"" w439 {
          tunnel: w440 -> [w450 w453]
          tunnel: [w450 w452] -> w446
          tunnel: w443 -> [_ w451]
          frame Default {
          }
          frame "Stopped" {
            n163 = call <vilib>:"Destroy.vi"("error in (no error)"=w453, "SMO"=w451) -> ("error out"=w452:errorcluster)  [unwired: 9 in]
          }
        }
        n164 = call <vilib>:"Add State(s) to Queue__jki_lib_state_machine.vi"("State(s) in (\"\")"=w449) -> ("States Out"=w448:string)  [unwired: 14 in]
      }
      frame "---------- Splash ----------" {
        # "Template Separator\n(You can make a copy of, or modify, this frame)"
        n165 = call <vilib>:"Add State(s) to Queue__jki_lib_state_machine.vi"("State(s) in (\"\")"=w458) -> ("States Out"=w457:string)  [unwired: 14 in]
      }
      frame "Splash: Set Status" {
        # "Your code here.\n(You can make a copy of, or modify, this frame)"
        n166 = property on="Splash Status" class="Str"(error in=w461, "Value"=w462) -> (error out=w460:errorcluster)  [unwired: 1 in, 1 out]
        n167 = call <vilib>:"Add State(s) to Queue__jki_lib_state_machine.vi"("State(s) in (\"\")"=w465) -> ("States Out"=w464:string)  [unwired: 14 in]
      }
      frame "Splash: 2" {
        # "Your code here.\n(You can make a copy of, or modify, this frame)"
        n168 = call <vilib>:"Add State(s) to Queue__jki_lib_state_machine.vi"("State(s) in (\"\")"=w470) -> ("States Out"=w469:string)  [unwired: 14 in]
      }
    }
  }
  "error out" <- w1
